vi "Shift Zero.vi"   [LabVIEW 2019, in "xy_utilities.lvlib"]
doc: "Given a fractional x value, interpolate a factional y value.\n\nWire data to the data input to determine the polymorphic instance to use or manually select the instance."
uses:
  xy_utilities.lvlib
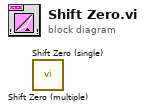
[diagram p0: block diagram]
diagram:
  n1 = call "Shift Zero (multiple).vi"() -> ()  [unwired: 10 in, 2 out]
  n2 = call "Shift Zero (single).vi"() -> ()  [unwired: 10 in, 2 out]
